vi "Get package_template_enum for Value.vi"(8 "error in (no error)":errorcluster, 10 "value in proto":i32, 11 "gRPC ID":T1) -> (0 "error out":errorcluster, 2 "value in LV":u32, 3 "gRPC ID Out":T1)   [LabVIEW 2024, in "Client Template.lvlib"]
uses:
  Client Template.lvlib
  gRPC lv Support/grpc-lvsupport/grpc-lvsupport.lvlib
  gRPC lv Support/grpc-lvsupport/grpcId.ctl
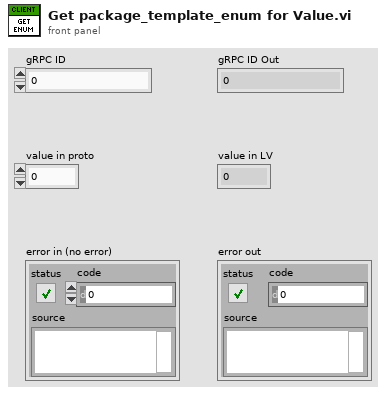
[diagram p1: front panel]
types:
  T1 = typedef "grpc-lvsupport.lvlib/grpcId.ctl" = u64
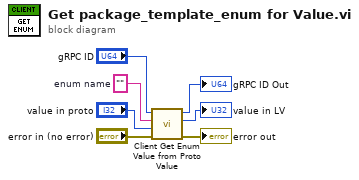
[diagram p0: block diagram]
diagram:
  w6 = ""  # enum name
  n1 = call "Client Get Enum Value from Proto Value.vi"("error in (no error)"="error in (no error)", "value in proto"="value in proto", "enum name"=w6, "gRPC ID in"="gRPC ID") -> ("error out"=→"error out":errorcluster, "value in LV"=→"value in LV":u32, "gRPC ID out"=→"gRPC ID Out":T1)  [unwired: 5 in]
